vi "Script Request and Wait For Reply Restore Timeout.vi"(8 "error in":errorcluster, 10 "VI":refnum<class "VI.lvclass">, 11 "Library":refnum<class "Library.lvclass">) -> (0 "error out":errorcluster)   [LabVIEW 2020, in "Panther Dashboard.lvlib"]
uses:
  Panther Dashboard.lvlib
  Class/Library/Library.lvclass
  C:/GitClones/PantherDashboard/src/LabVIEW/Panther Dashboard/Class/LabVIEWItem/LabVIEWItem.lvclass
  Class/VI/VI.lvclass
  <vilib>/Utility/traverseref.llb/TRef TravTarget.ctl
  Class/LabVIEWItem/LabVIEWItem.lvclass/LabVIEWItem.ctl
  Class/LabVIEWItem/Read Item Path.vi
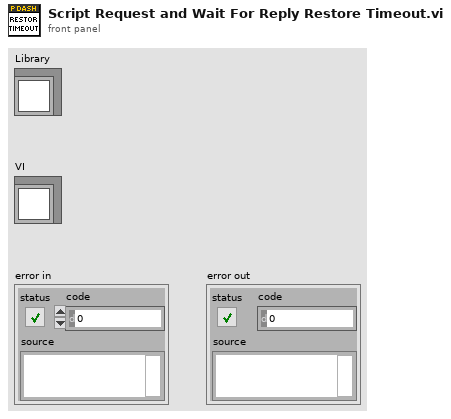
[diagram p1: front panel]
types:
  T1 = typedef "TRef TravTarget.ctl" = enum16{"FP", "BD", "Other"}
  T2 = typedef "LVPositionTypeDef.ctl" = cluster{"Left":i32, "Top":i32}
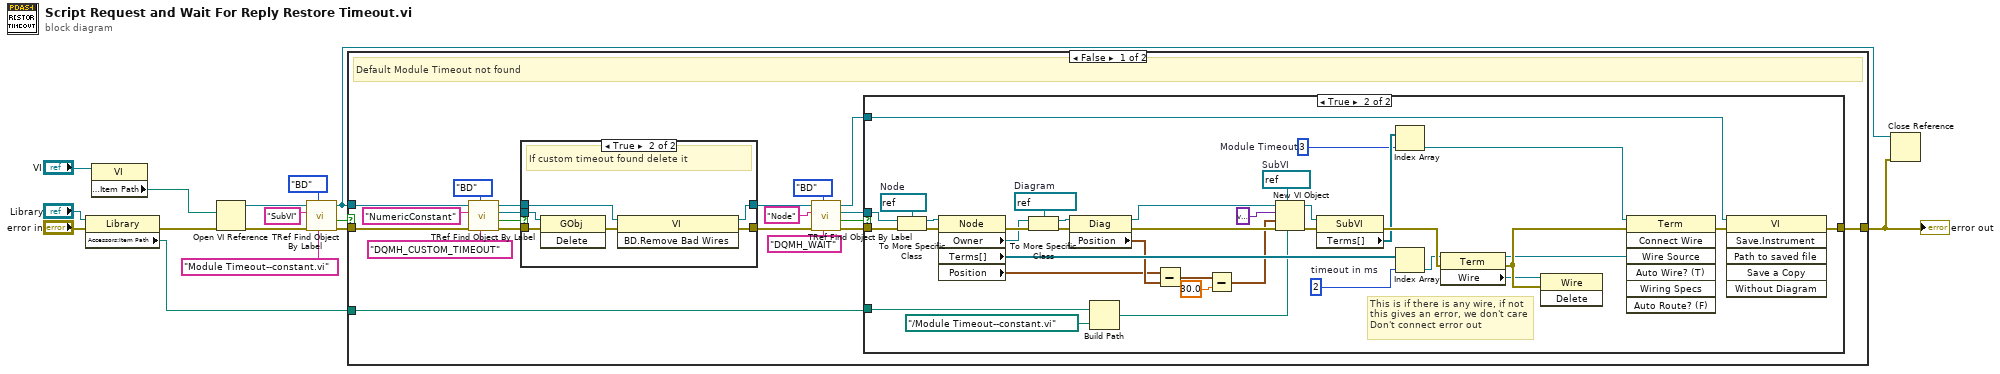
[diagram p0: block diagram]
diagram:
  n1 = property class="Library"(reference="Library", error in="error in") -> (error out=w14:errorcluster, "Accessors:Item Path"=w6:path)  [unwired: 1 out]
  n2 = property class="VI"(reference="VI") -> ("Accessors:Item Path"=w3:path)  [unwired: 1 in, 2 out]
  n3 = Open VI Reference(vi path=w3, error in (no error)=w14) -> (vi reference=w2:refnum<vi>, error out=w12:errorcluster)  [unwired: 4 in]
  n4 = call <vilib>:"TRef Find Object By Label.vi"("Label"="Module Timeout--constant.vi", "Traverse Target"=TRef_TravTarget."BD", "error in (no error)"=w12, "Class Name"="SubVI", "VI Ref"=w2) -> ("error out"=w13:errorcluster, "Found?"=w7:bool, "dup VI Ref"=w1:refnum<vi>)  [unwired: 3 in, 1 out]
  n5 = case shown="False" w7 {
    tunnel: [w35 w82] -> w11
    tunnel: w13 -> [w32 w82]
    tunnel: w1 -> [w23 _]
    tunnel: w6 -> [w16 _]
    frame False {
      # "Default Module Timeout not found"
      n6 = call <vilib>:"TRef Find Object By Label.vi"("Label"="DQMH_CUSTOM_TIMEOUT", "Traverse Target"=TRef_TravTarget."BD", "error in (no error)"=w32, "Class Name"="NumericConstant", "VI Ref"=w23) -> ("error out"=w31:errorcluster, "Found?"=w18:bool, "Found Obj Ref"=w24:refnum<vi>, "dup VI Ref"=w22:refnum<vi>)  [unwired: 3 in]
      n7 = case shown="True" w18 {
        tunnel: [w75 w81] -> w33
        tunnel: [w74 w78] -> w25
        tunnel: w24 -> [_ w77]
        tunnel: w31 -> [w75 w79]
        tunnel: w22 -> [w74 w76]
        frame False {
        }
        frame True {
          # "If custom timeout found delete it"
          n8 = invoke class="GObj" method="Delete"(reference=w77, error in=w79) -> (error out=w80:errorcluster)  [unwired: 1 in, 2 out]
          n9 = invoke class="VI" method="BD.Remove Bad Wires"(reference=w76, error in=w80) -> (reference out=w78:refnum<vi>, error out=w81:errorcluster)  [unwired: 1 in, 1 out]
        }
      }
      n10 = call <vilib>:"TRef Find Object By Label.vi"("Label"="DQMH_WAIT", "Traverse Target"=TRef_TravTarget."BD", "error in (no error)"=w33, "Class Name"="Node", "VI Ref"=w25) -> ("error out"=w34:errorcluster, "Found?"=w27:bool, "Found Obj Ref"=w28:refnum<vi>, "dup VI Ref"=w17:refnum<vi>)  [unwired: 3 in]
      n11 = case shown="True" w27 {
        tunnel: w28 -> [_ w63]
        tunnel: w34 -> [w36 w73]
        tunnel: [w36 w68] -> w35
        tunnel: w17 -> [_ w51]
        tunnel: w16 -> [_ w40]
        frame False {
        }
        frame True {
          w47 = refnum<vi> refnum  # Diagram
          w54 = 3  # Module Timeout
          w58 = refnum<vi> refnum  # SubVI
          w60 = 2  # timeout in ms
          w62 = refnum<vi> refnum  # Node
          # "This is if there is any wire, if not\nthis gives an error, we don't care\nDon't connect error out"
          n12 = To More Specific Class(target class=w62, reference=w63, error in=w73) -> (specific class reference=w61:refnum<vi>, error out=w72:errorcluster)
          n13 = property class="Node"(reference=w61, error in=w72) -> (error out=w71:errorcluster, "Owner"=w49:refnum<vi>, "Terms[]"=w57:refnum<vi>[], "Position"=w44:T2)  [unwired: 1 out]
          n14 = To More Specific Class(target class=w47, reference=w49, error in=w71) -> (specific class reference=w48:refnum<vi>, error out=w66:errorcluster)
          n15 = property class="Diag"(reference=w48, error in=w66) -> (reference out=w50:refnum<vi>, error out=w67:errorcluster, "Position"=w46:T2)
          n16 = Build Path(base path=w40, name or relative path=path "../Module Timeout--constant.vi") -> (appended path=w39:path)
          n17 = Subtract(x=w44, y=w46) -> (x-y=w45:T2)
          n18 = Subtract(x=w45, y=30.0) -> (x-y=w43:cluster{"Left":dbl, "Top":dbl})
          n19 = New VI Object(vi object class=w58, owner refnum=w50, style=variant, position/next to=w43, 6:w39, 8:w67) -> (object refnum=w56:refnum<vi>, 0:w70:errorcluster)  [unwired: 2 in]
          n20 = property class="SubVI"(reference=w56, error in=w70) -> (error out=w65:errorcluster, "Terms[]"=w55:refnum<vi>[])  [unwired: 1 out]
          n21 = Index Array(array=w55, index=w54) -> (element=w53:refnum<vi>)
          n22 = Index Array(array=w57, index=w60) -> (element=w52:refnum<vi>)
          n23 = property class="Term"(reference=w52, error in=w65) -> (reference out=w38:refnum<vi>, error out=w64:errorcluster, "Wire"=w37:refnum<vi>)
          n24 = invoke class="Wire" method="Delete"(reference=w37, error in=w64) -> ()  [unwired: 1 in, 3 out]
          n25 = invoke class="Term" method="Connect Wire"(reference=w53, error in=w64, "Wire Source"=w38) -> (error out=w69:errorcluster)  [unwired: 4 in, 6 out]
          n26 = invoke class="VI" method="Save.Instrument"(reference=w51, error in=w69) -> (error out=w68:errorcluster)  [unwired: 4 in, 5 out]
        }
      }
    }
    frame True {
      # "Request and wait for Reply already has the Module's Default Timeout"
    }
  }
  "error out" <- w11
  n27 = Close Reference(reference=w1, error in (no error)=w11) -> ()  [unwired: 1 out]
